vi "endLine.vi"(10 "scan info":T2, 11 "reader status in":T1) -> (3 "reader status out":T1)   [LabVIEW 2010]
panel:
  out "error out":errorcluster
  in  "error in (no error)":errorcluster
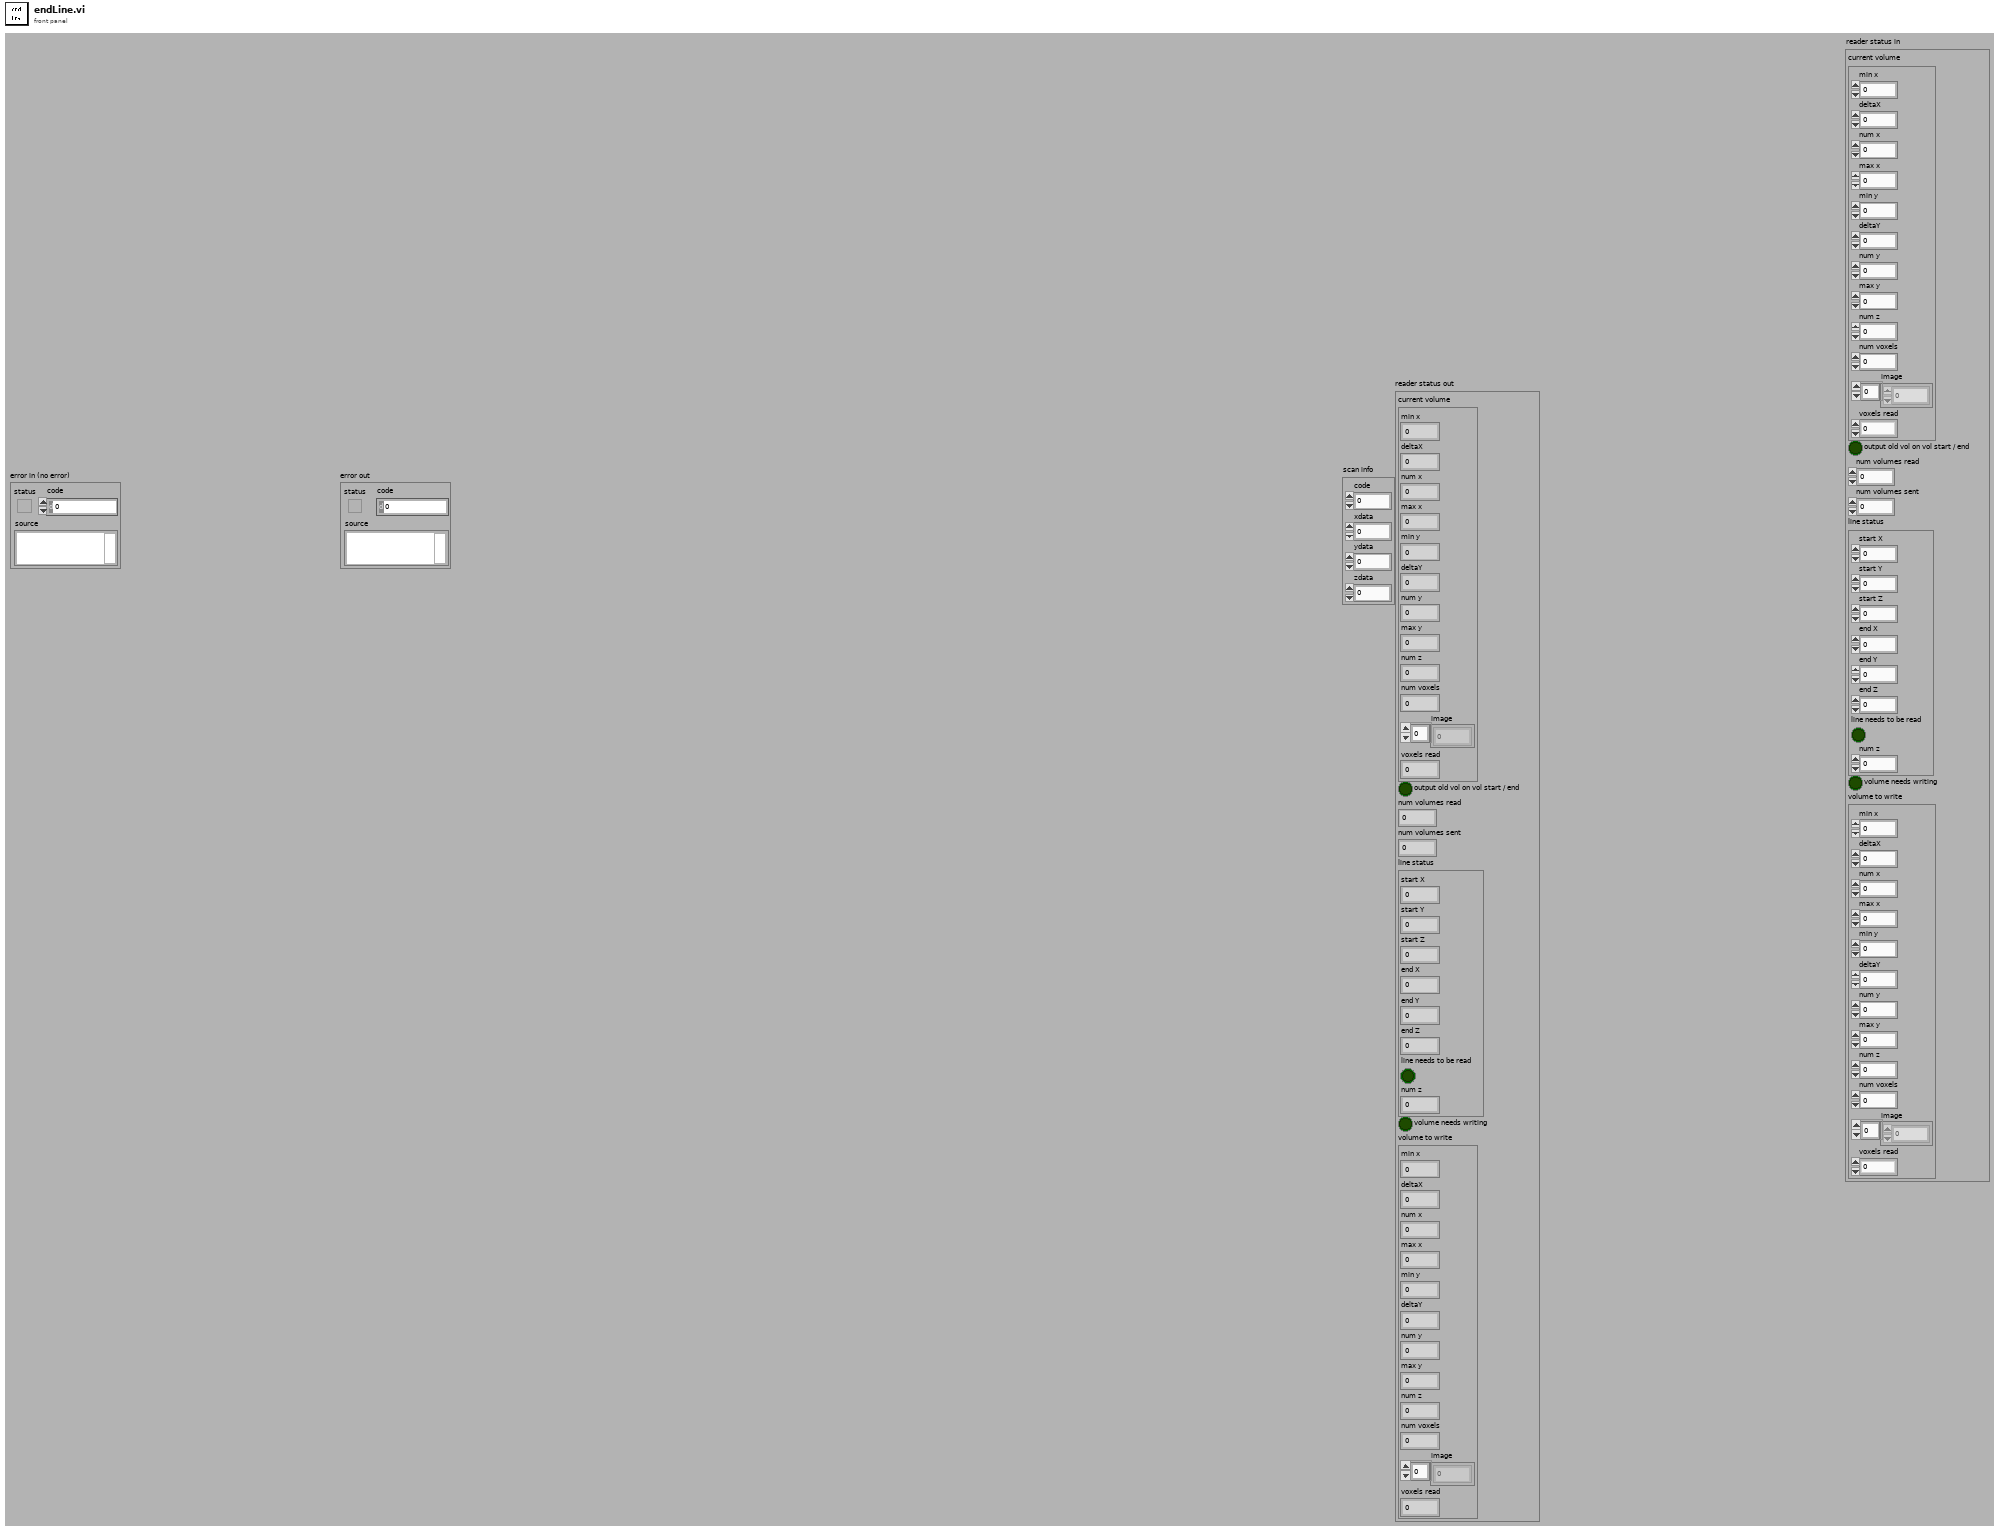
[diagram p1: front panel]
types:
  T1 = cluster{"current volume":cluster{"min x":i16, "deltaX":dbl, "num x":u32, "max x":i16, "min y":i16, "deltaY":dbl, "num y":u32, "max y":i16, "num z":u32, "num voxels":u32, "image":u32[], "voxels read":u32}, "output old vol on vol start / end":bool, "num volumes read":u32, "num volumes sent":u32, "line status":cluster{"start X":i16, "start Y":i16, "start Z":i16, "end X":i16, "end Y":i16, "end Z":i16, "line needs to be read":bool, "num z":u8}, "volume needs writing":bool, "volume to write":cluster{"min x":i16, "deltaX":dbl, "num x":u32, "max x":i16, "min y":i16, "deltaY":dbl, "num y":u32, "max y":i16, "num z":u32, "num voxels":u32, "image":u32[], "voxels read":u32}}
  T2 = cluster{"code":i32, "xdata":i32, "ydata":i32, "zdata":i32}
  T3 = enum16{"NONE", "VOLUME_START", "LINE_START", "LINE_END", "VOLUME_END"}
  T4 = cluster{"start X":i16, "start Y":i16, "start Z":i16, "end X":i16, "end Y":i16, "end Z":i16, "line needs to be read":bool, "num z":u8}
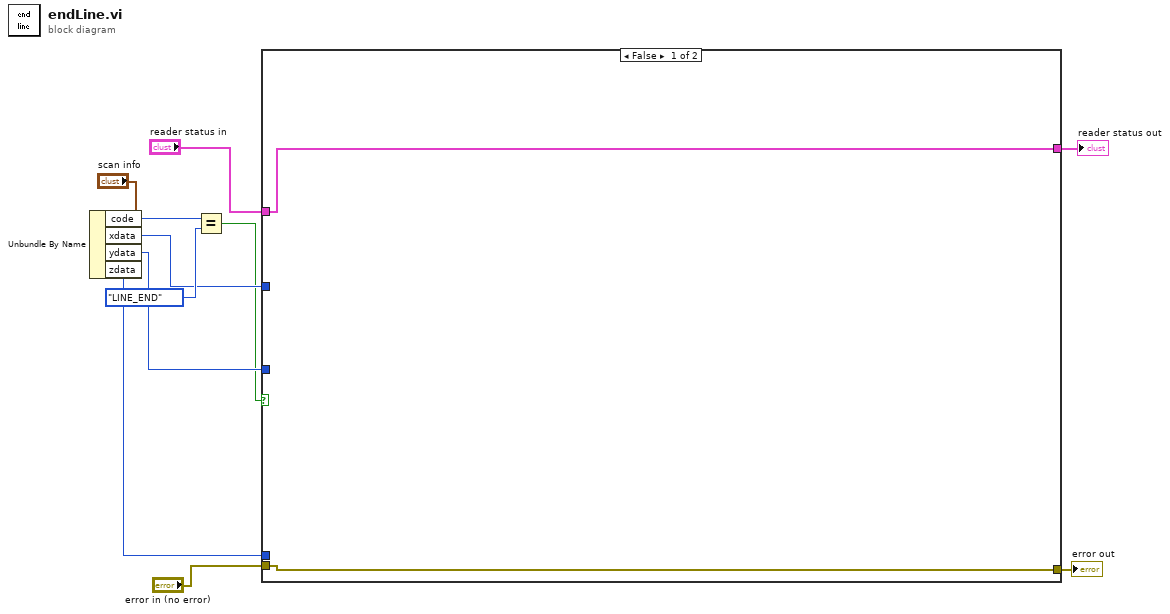
[diagram p0: block diagram]
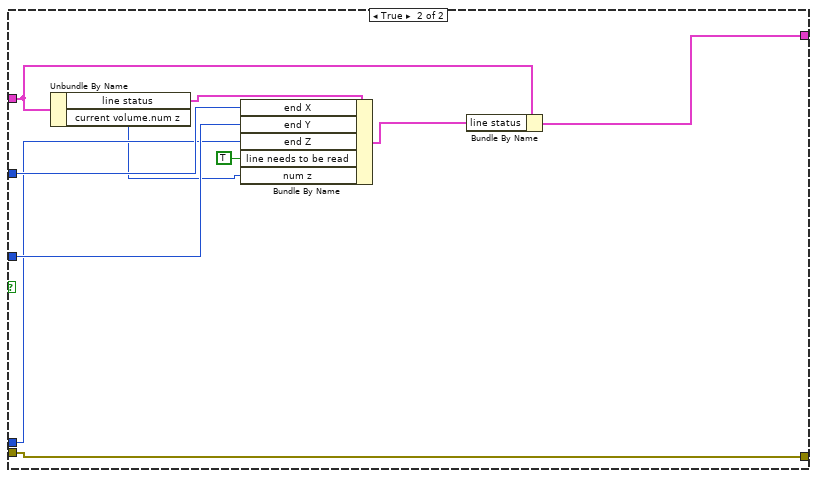
[diagram p2: hidden frame]
diagram:
  n1 = Unbundle By Name("scan info") -> ("code"=w10:i32, "xdata"=w8:i32, "ydata"=w7:i32, "zdata"=w6:i32)
  n2 = Equal?(x=w10, y=T3."LINE_END" ("message")) -> (x = y?=w4:bool)
  n3 = case shown="False" w4 {
    tunnel: w8 -> [_ w22]
    tunnel: w7 -> [_ w21]
    tunnel: w6 -> [_ w20]
    tunnel: "reader status in" -> [w13 w18]
    tunnel: [w13 w16] -> w3
    tunnel: "error in (no error)" -> [w12 w14]
    tunnel: [w12 w14] -> w1
    frame False {
    }
    frame True {
      n4 = Unbundle By Name(w18) -> ("line status"=w23:T4, "current volume.num z"=w15:u32)
      n5 = Bundle By Name(cluster=w23, "end X"=w22, "end Y"=w21, "end Z"=w20, "line needs to be read"=TRUE, "num z"=w15) -> (w17:T4)
      n6 = Bundle By Name(cluster=w18, "line status"=w17) -> (w16:T1)
    }
  }
  "reader status out" <- w3
  "error out" <- w1
